vi "Parse.vi"(8 "error in (no error)":errorcluster, 11 "Transform.Rotate in":refnum<class "Transform.Rotate.lvclass">) -> (0 "error out":errorcluster, 3 "Transform.Rotate out":refnum<class "Transform.Rotate.lvclass">)   [LabVIEW 2019, in "Transform.Rotate.lvclass"]
uses:
  Transform.Rotate.lvclass
  C:/Users/Albro/Documents/GitHub/AFM-Lithography/lvsrc/Classes/Parse/Transform/Transform.lvclass
  Transform/Transform.lvclass/Transform.ctl
  Transform/Transform.lvclass
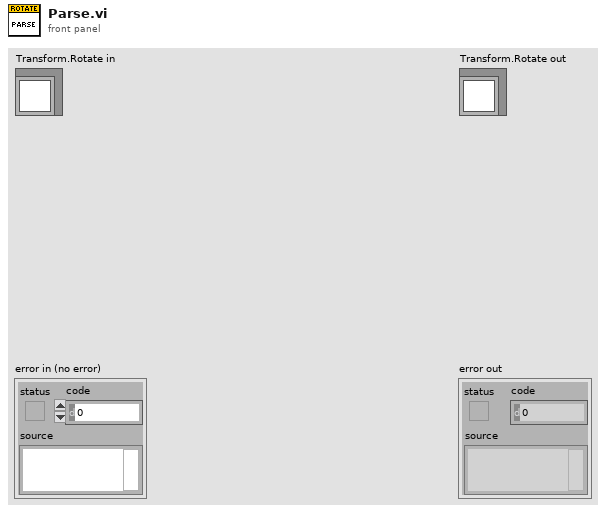
[diagram p1: front panel]
types:
  T1 = typedef "NI_Matrix.lvlib/RealMatrix.ctl" = dbl[][]
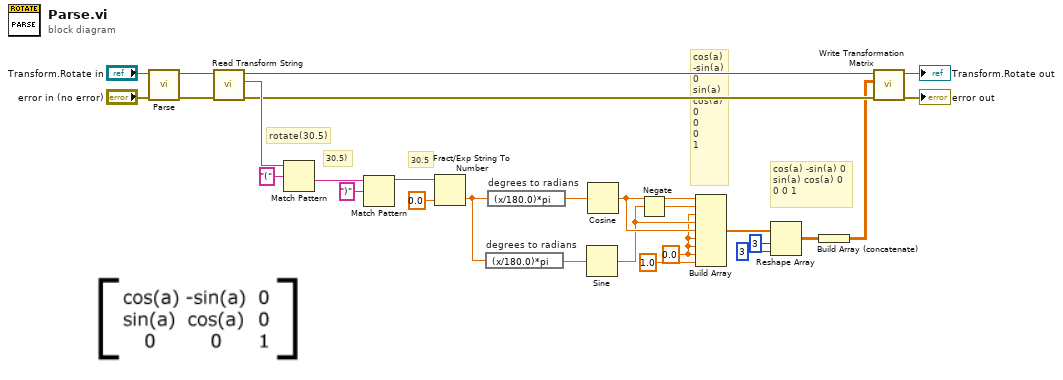
[diagram p0: block diagram]
diagram:
  w14 = 0.0 ("element")
  # "cos(a) -sin(a) 0\nsin(a) cos(a) 0\n0 0 1"
  # "cos(a)\n-sin(a)\n0\nsin(a)\ncos(a)\n0\n0\n0\n1"
  # "30.5"
  # "30.5)"
  # "rotate(30.5)"
  n1 = call-parent "Parse.vi"("error in (no error)"="error in (no error)", "Transform in"="Transform.Rotate in") -> ("error out"=w24:errorcluster, "Transform out"=w25:refnum<class "Transform.Rotate.lvclass">)  [unwired: 8 in]
  n2 = call "Read Transform String.vi"("error in (no error)"=w24, "Transform in"=w25) -> ("error out"=w3:errorcluster, "Transform String"=w6:string, "Transform out"=w5:refnum<class "Transform.Rotate.lvclass">)  [unwired: 7 in]
  n3 = Match Pattern(string=w6, regular expression="(") -> (after substring=w22:string)  [unwired: 1 in, 3 out]
  n4 = Match Pattern(string=w22, regular expression=")") -> (before substring=w20:string)  [unwired: 1 in, 3 out]
  n5 = Fract/Exp String To Number(string=w20, default (0 dbl)=0.0 ("default (0 DBL)")) -> (number=w12:dbl)  [unwired: 2 in, 1 out]
  n6 = expression code="(x/180.0)*pi" "degrees to radians"(w12) -> (w11:dbl)
  n7 = expression code="(x/180.0)*pi" "degrees to radians"(w12) -> (w13:dbl)
  n8 = Sine(x=w11) -> (sin(x)=w16:dbl)
  n9 = Cosine(x=w13) -> (cos(x)=w17:dbl)
  n10 = Negate(x=w16) -> (-x=w18:dbl)
  n11 = Build Array(w17, w18, w14, w16, w17, w14, w14, w14, 1.0 ("element")) -> (w10:dbl[])
  n12 = Reshape Array(w10, 3 ("dimension size"), 3 ("dimension size")) -> (w7:dbl[][])
  n13 = Build Array (concatenate)(w7) -> (w1:T1)
  n14 = call "Write Transformation Matrix.vi"("error in (no error)"=w3, "Real Matrix"=w1, "Transform in"=w5) -> ("error out"=→"error out":errorcluster, "Transform out"=→"Transform.Rotate out":refnum<class "Transform.Rotate.lvclass">)  [unwired: 7 in]
